vi "Generate-b.vi"(11 "Error in":errorcluster) -> (15 "error out":errorcluster)   [LabVIEW 2020]
doc: "This VI will generate numeric data and transfers to acquire VI with the help of LV2"
uses:
  Typedefs/LV2 numeric.ctl
panel:
  in  "Stop":bool
  # "GENERATE"
  # "This VI will generate random numbers and populate\nit to the acquire VI"
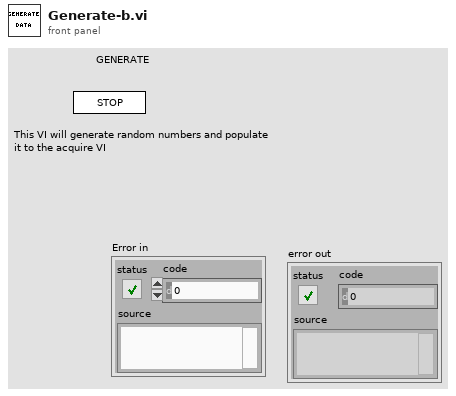
[diagram p1: front panel]
types:
  T1 = typedef "LV2 numeric.ctl" = enum16{"Initialize", "Read", "Write"}
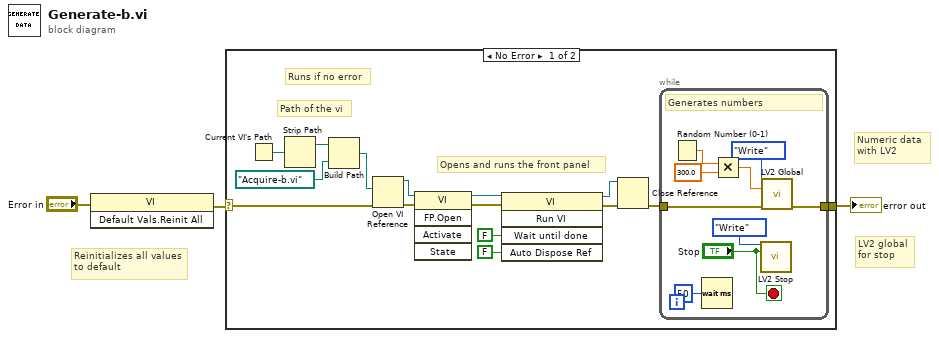
[diagram p0: block diagram]
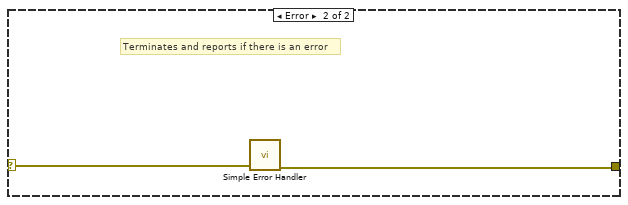
[diagram p2: hidden frame]
diagram:
  # "LV2 global\nfor stop"
  # "Numeric data\nwith LV2"
  # "Reinitializes all values\nto default"
  n1 = invoke class="VI" method="Default Vals.Reinit All"(error in="Error in") -> (error out=w2:errorcluster)  [unwired: 2 in, 2 out]
  n2 = case shown="No Error" w2 {
    selector: w2 -> [w11 w28]
    tunnel: [w10 w27] -> w1
    frame No Error {
      # "Opens and runs the front panel"
      # "Path of the vi"
      # "Runs if no error"
      n3 = Current VI's Path() -> (path=w17:path)
      n4 = Strip Path(path=w17) -> (stripped path=w16:path)  [unwired: 1 out]
      n5 = Build Path(base path=w16, name or relative path=path "Acquire-b.vi") -> (appended path=w14:path)
      n6 = Open VI Reference(vi path=w14, error in (no error)=w11) -> (vi reference=w12:refnum<vi>, error out=w13:errorcluster)  [unwired: 4 in]
      n7 = invoke class="VI" method="FP.Open"(reference=w12, error in=w13) -> (reference out=w7:refnum<vi>, error out=w8:errorcluster)  [unwired: 3 in, 3 out]
      n8 = invoke class="VI" method="Run VI"(reference=w7, error in=w8, "Wait until done"=FALSE ("Wait Until Done"), "Auto Dispose Ref"=FALSE ("Auto Dispose Reference")) -> (reference out=w4:refnum<vi>, error out=w9:errorcluster)  [unwired: 1 in, 3 out]
      n9 = Close Reference(reference=w4) -> ()  [unwired: 1 in, 1 out]
      n10 = while {
        tunnel: [w22] -> w10
        tunnel: w9 -> [w23]
        stop <- "Stop" stop-if-true
        # "Generates numbers"
        n11 = Random Number (0-1)() -> (number: 0 to 1=w26:dbl)
        n12 = Wait (ms)(milliseconds to wait=u32 50) -> ()  [unwired: 1 out]
        n13 = Multiply(x=w26, y=300.0) -> (x*y=w24:dbl)
        n14 = call "LV2 Stop.vi"("Operation"=enum16{"Initialize", "Write", "Stop"}."Write", "Stop"="Stop") -> ()  [unwired: 12 in, 2 out]
        n15 = call "LV2 Global.vi"("Operation"=LV2_numeric."Write", "Numeric Input"=w24, "Error in"=w23) -> ("Error out"=w22:errorcluster)  [unwired: 11 in, 1 out]
      }
    }
    frame Error {
      # "Terminates and reports if there is an error"
      n16 = call <vilib>:"Simple Error Handler.vi"("error in (no error)"=w28) -> ("error out"=w27:errorcluster)  [unwired: 4 in, 4 out]
    }
  }
  "error out" <- w1
